vi "E8267D ModulationEn.vi"(0 "VISA Rsrc":refnum<visa-resource-name>="GPIB0::12::INSTR", 5 "Modulation En":bool, 11 "error in (no error)":errorcluster, 13 "Set?(F)":bool) -> (4 "VISA Rsrc Out":refnum<visa-resource-name>="GPIB0::12::INSTR", 6 "Enabled":bool, 15 "error out":errorcluster)   [LabVIEW 2019]
doc: "Ce VI écrit les paramètres de la zone de contrôle spécifiée dans le contrôlleur"
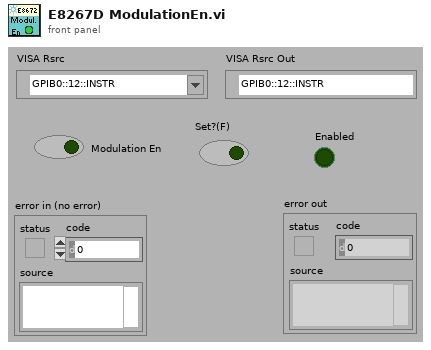
[diagram p1: front panel]
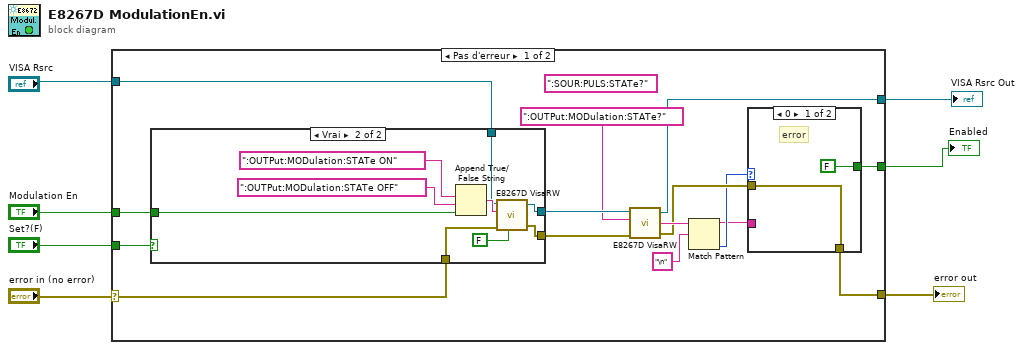
[diagram p0: block diagram]
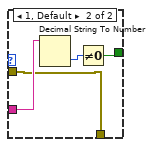
[diagram p3: hidden frame]
diagram:
  n1 = case shown="Pas d'erreur" "error in (no error)" {
    selector: "error in (no error)" -> [w12 w41]
    tunnel: "VISA Rsrc" -> [w10 w40]
    tunnel: [w19 w41] -> w6
    tunnel: [w22 w40] -> w4
    tunnel: "Set?(F)" -> [w13 _]
    tunnel: [w15 _] -> w2
    tunnel: "Modulation En" -> [w14 _]
    frame No Error {
      (unwired) ":SOUR:PULS:STATe?" ("true string")
      n2 = case shown="Vrai" w13 {
        tunnel: w14 -> [_ w30]
        tunnel: w12 -> [w24 w29]
        tunnel: [w24 w28] -> w11
        tunnel: w10 -> [w23 w26]
        tunnel: [w23 w25] -> w9
        frame False {
        }
        frame True {
          n3 = Append True/False String(1:w30, 2:":OUTPut:MODulation:STATe OFF" ("true string"), 3:":OUTPut:MODulation:STATe ON" ("true string")) -> (0:w31:string)  [unwired: 1 in]
          n4 = call <userlib>:"E8267D VisaRW.vi"("Lecture?(T)"=FALSE, "error in (no error)"=w29, "ChaineCom"=w31, "VISA Rsrc"=w26) -> ("error out"=w28:errorcluster, "VISA Rsrc Out"=w25:refnum<visa-resource-name>)  [unwired: 3 in, 2 out]
        }
      }
      n5 = call <userlib>:"E8267D VisaRW.vi"("error in (no error)"=w11, "ChaineCom"=":OUTPut:MODulation:STATe?" ("true string"), "VISA Rsrc"=w9) -> ("error out"=w20:errorcluster, "ChaineRep"=w21:string, "VISA Rsrc Out"=w22:refnum<visa-resource-name>)  [unwired: 4 in, 1 out]
      n6 = Match Pattern(string=w21, regular expression="\n" ("expression régulière")) -> (before substring=w16:string, offset past match=w17:i32)  [unwired: 1 in, 2 out]
      n7 = case shown="0" w17 {
        tunnel: w20 -> [w35 w36]
        tunnel: [w35 w36] -> w19
        tunnel: w16 -> [_ w39]
        tunnel: [FALSE w38] -> w15
        frame 0 {
          # "error"
        }
        frame 1, Default {
          n8 = Decimal String To Number(string=w39) -> (number=w37:i32)  [unwired: 2 in, 1 out]
          n9 = Not Equal To 0?(x=w37) -> (x != 0?=w38:bool)
        }
      }
    }
    frame Error {
    }
  }
  "error out" <- w6
  "VISA Rsrc Out" <- w4
  "Enabled" <- w2
